vi "Read Enabled Controllers.vi"(8 "error in (no error)":errorcluster, 11 "Num Array in":refnum<class "Num Array.lvclass">) -> (0 "error out":errorcluster, 2 "Enabled Controllers":string[](array[string]), 3 "Num Array out":refnum<class "Num Array.lvclass">)   [LabVIEW 2018, in "Num Array.lvclass"]
doc: "NI Analog Out.lvclass:Read Enabled Channels.vi\n\nThis VI returns the list of channel names that are enabled for the NI Analog Out class..\n\nInstrument Communication Module Version 1.0\nOctober, 2020 Original Code Consulting Davita Bird\n www.originalcode.com"
uses:
  Num Array.lvclass
  Num Array.lvclass/Num Array.ctl
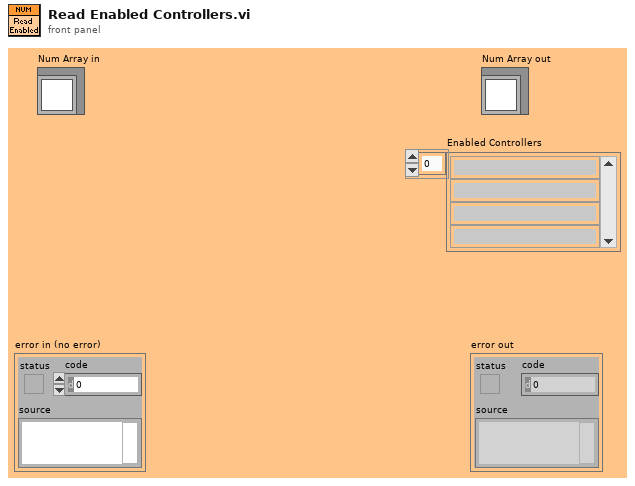
[diagram p1: front panel]
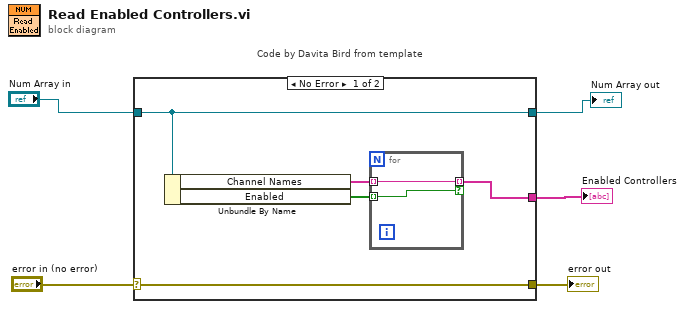
[diagram p0: block diagram]
diagram:
  n1 = case "Code by Davita Bird from template" shown="No Error" "error in (no error)" {
    selector: "error in (no error)" -> [w10 w13]
    tunnel: [w10 w13] -> w4
    tunnel: [w9 w14] -> w1
    tunnel: "Num Array in" -> [w9 w14]
    tunnel: [w6 _] -> w3
    frame No Error {
      n2 = Unbundle By Name(w9) -> ("Channel Names"=w8:string[], "Enabled"=w7:bool[])
      n3 = for {
        tunnel: [w12] -> w6 mode=indexing if=w11
        tunnel: w8 -> [w12] mode=indexing
        tunnel: w7 -> [w11] mode=indexing
      }
    }
    frame Error {
    }
  }
  "error out" <- w4
  "Enabled Controllers" <- w3
  "Num Array out" <- w1
